vi "Calc R2.vi"(2 "Clean Data":bool, 3 "Fit":dbl[](array[numeric]), 4 "Data":dbl[](array[numeric])) -> (1 "R²":dbl)   [LabVIEW 2010]
uses:
  <vilib>/Analysis/NI_AALBase.lvlib
panel:
  out "x-y 2":dbl[](array[numeric])
  out "sum 2":dbl
  out "sum":dbl
  out "x-y":dbl[](array[numeric])
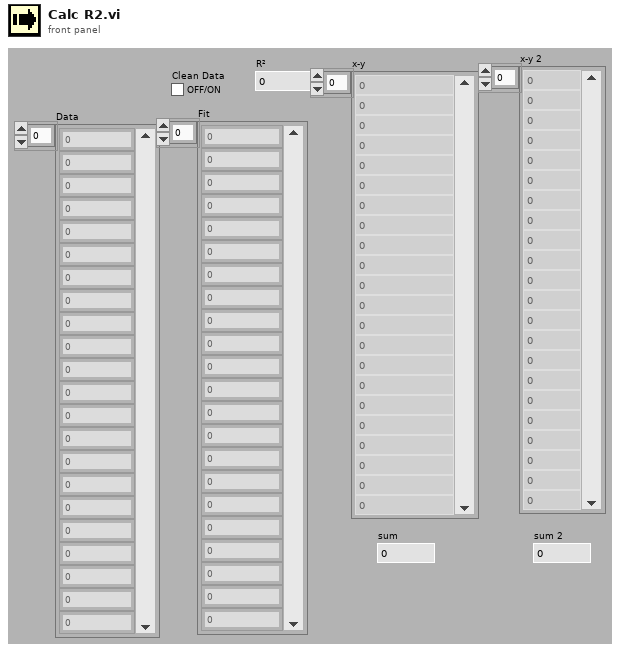
[diagram p1: front panel]
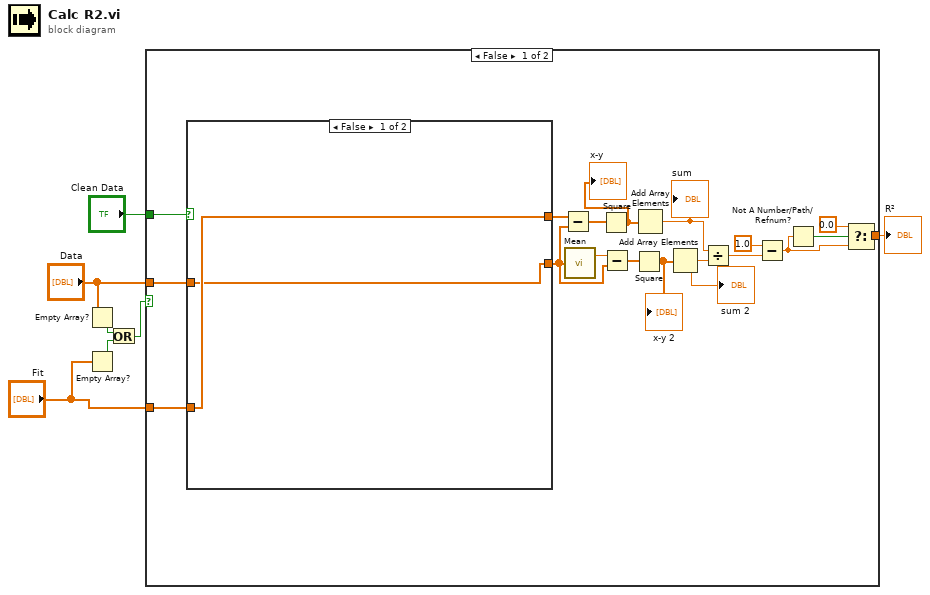
[diagram p0: block diagram]
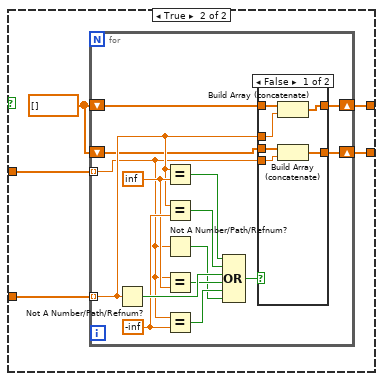
[diagram p2: hidden frame]
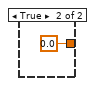
[diagram p4: hidden frame]
diagram:
  n1 = Empty Array?(array="Data") -> (empty?=w3:bool)
  n2 = Empty Array?(array="Fit") -> (empty?=w2:bool)
  n3 = Or(x=w3, y=w2) -> (x .or. y?=w1:bool)
  n4 = case shown="False" w1 {
    tunnel: [w15 0.0 ("t")] -> w7
    tunnel: "Clean Data" -> [w14 _]
    tunnel: "Fit" -> [w13 _]
    tunnel: "Data" -> [w11 _]
    frame False {
      n5 = case shown="False" w14 {
        tunnel: w13 -> [w27 w31]
        tunnel: [w27 w30] -> w12
        tunnel: w11 -> [w26 w32]
        tunnel: [w26 w29] -> w10
        frame False {
        }
        frame True {
          w28 = dbl[] []
          n6 = for {
            tunnel: w32 -> [w37] mode=indexing
            tunnel: w31 -> [w38] mode=indexing
            shift-right: [w36] -> w30
            shift-left: w28 -> [w35]
            shift-right: [w34] -> w29
            shift-left: w28 -> [w33]
            w44 = -inf
            w43 = inf
            n7 = Not A Number/Path/Refnum?(number/path/refnum=w38) -> (NaN/Path/Refnum?=w47:bool)
            n8 = Equal?(x=w38, y=w43) -> (x = y?=w45:bool)
            n9 = Equal?(x=w38, y=w44) -> (x = y?=w46:bool)
            n10 = Not A Number/Path/Refnum?(number/path/refnum=w37) -> (NaN/Path/Refnum?=w40:bool)
            n11 = Equal?(x=w37, y=w43) -> (x = y?=w42:bool)
            n12 = Equal?(x=w37, y=w44) -> (x = y?=w41:bool)
            n13 = Compound Arithmetic op=OR(w45, w46, w47, w42, w41, w40) -> (w39:bool)
            n14 = case shown="False" w39 {
              tunnel: w38 -> [w53 _]
              tunnel: w37 -> [w50 _]
              tunnel: [w52 w55] -> w36
              tunnel: w35 -> [w51 w55]
              tunnel: [w49 w54] -> w34
              tunnel: w33 -> [w48 w54]
              frame False {
                n15 = Build Array (concatenate)(w51, w53) -> (w52:dbl[])
                n16 = Build Array (concatenate)(w48, w50) -> (w49:dbl[])
              }
              frame True {
              }
            }
          }
        }
      }
      n17 = Subtract(x=w12, y=w10) -> (x-y=w21:dbl[])
      n18 = call <vilib>:"Mean.vi"("X"=w10) -> ("mean"=w19:dbl)  [unwired: 1 out]
      n19 = Square(x=w21) -> (x^2=w8:dbl[])
      "x-y" <- w8
      n20 = Subtract(x=w19, y=w10) -> (x-y=w20:dbl[])
      n21 = Square(x=w20) -> (x^2=w9:dbl[])
      "x-y 2" <- w9
      n22 = Add Array Elements(numeric array=w8) -> (sum=w25:dbl)
      "sum" <- w25
      n23 = Add Array Elements(numeric array=w9) -> (sum=w24:dbl)
      "sum 2" <- w24
      n24 = Divide(x=w25, y=w24) -> (x/y=w22:dbl)
      n25 = Subtract(x=1.0, y=w22) -> (x-y=w17:dbl)
      n26 = Not A Number/Path/Refnum?(number/path/refnum=w17) -> (NaN/Path/Refnum?=w18:bool)
      n27 = Select(t=0.0, s=w18, f=w17) -> (s? t:f=w15:dbl)
    }
    frame True {
    }
  }
  "R²" <- w7
